vi "load_dictionary_xml.vi"(7 "unit_dictionary in":variant, 8 "error in (no error)":errorcluster, 10 "symbols []":string[](array[string]), 11 "xml_path":path) -> (0 "error out":errorcluster, 3 "unit_dictionary":variant)   [LabVIEW 2015, in "lv-unit-conversion.lvlib"]
uses:
  lv-unit-conversion.lvlib
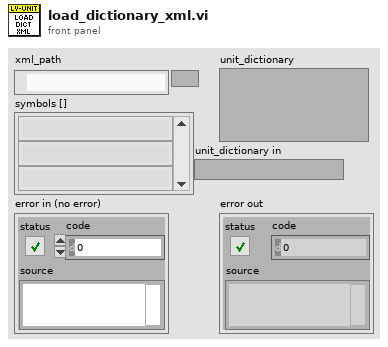
[diagram p1: front panel]
types:
  T1 = typedef "lv-unit-conversion.lvlib/unit.ctl" = cluster{"symbol":string, "name":string, "dimension":string, "is_si_unit":bool, "category":string, "base_unit":string, "conversion_reference":string, "is_exact":bool, "a":dbl, "b":dbl, "c":dbl, "d":dbl, "underlying_def":string, "description":string}
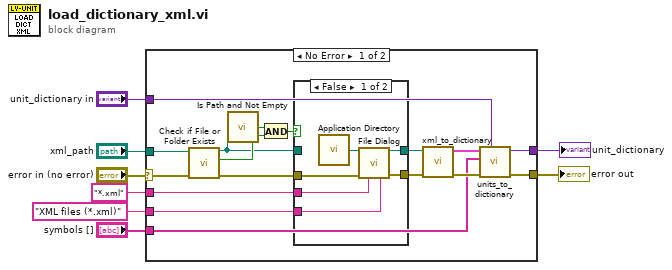
[diagram p0: block diagram]
diagram:
  n1 = case shown="No Error" "error in (no error)" {
    selector: "error in (no error)" -> [w22 w34]
    tunnel: "*.xml" ("pattern (all files)") -> [w25 _]
    tunnel: "XML files (*.xml)" ("pattern label") -> [w24 _]
    tunnel: "xml_path" -> [w23 _]
    tunnel: [w11 w34] -> w4
    tunnel: [w12 _] -> w3
    tunnel: "symbols []" -> [w10 _]
    tunnel: "unit_dictionary in" -> [w9 _]
    frame No Error {
      n2 = call <vilib>:"Check if File or Folder Exists.vi"("error in (no error)"=w22, "path"=w23) -> ("error out"=w21:errorcluster, "file or folder exists?"=w20:bool, "dup path"=w17:path)  [unwired: 7 in]
      n3 = call <vilib>:"Is Path and Not Empty.vi"("path"=w17) -> ("Is Path and Not Empty?"=w19:bool)  [unwired: 4 in]
      n4 = And(x=w19, y=w20) -> (x .and. y?=w18:bool)
      n5 = case shown="False" w18 {
        tunnel: w25 -> [w31 _]
        tunnel: w24 -> [w30 _]
        tunnel: [w29 w33] -> w16
        tunnel: [w28 w32] -> w15
        tunnel: w21 -> [w27 w32]
        tunnel: w17 -> [_ w33]
        frame False {
          n6 = call <vilib>:"Application Directory.vi"() -> ("Application Directory"=w26:path)
          n7 = call "File Dialog"("start path"=w26, "error in"=w27, "pattern (all files)"=w31, "pattern label"=w30) -> ("selected path"=w29:path, "error out"=w28:errorcluster)  [unwired: 8 in, 2 out]
        }
        frame True {
        }
      }
      n8 = call "xml_to_dictionary.vi"("error in (no error)"=w15, "XML File Path"=w16) -> ("error out"=w13:errorcluster, "units []"=w14:T1[])  [unwired: 8 in]
      n9 = call "units_to_dictionary.vi"("unit_dictionary in"=w9, "error in (no error)"=w13, "symbols []"=w10, "units []"=w14) -> ("error out"=w11:errorcluster, "unit_dictionary out"=w12:variant)  [unwired: 6 in]
    }
    frame Error {
    }
  }
  "error out" <- w4
  "unit_dictionary" <- w3
